vi "FilterSettings.Reset.vi"(8 "error in (no error)":errorcluster, 10 "Default Filter":T1, 11 "FilterDVR.Ref":refnum<data-value>) -> (0 "error out":errorcluster, 3 "Filter":T1)   [LabVIEW 2025, in "bus_monitor_server_do.lvlib"]
uses:
  bus_monitor_server_do.lvlib
  bus_monitor_server/RPC Messages/ni_bus_monitor_api_FilterInfo.ctl
  bus_monitor_server/RPC Messages/ni_bus_monitor_api_DirectionFilter.ctl
  bus_monitor_server/RPC Messages/ni_bus_monitor_api_FrameFilter.ctl
  bus_monitor_server/bus_monitor_server.lvlib
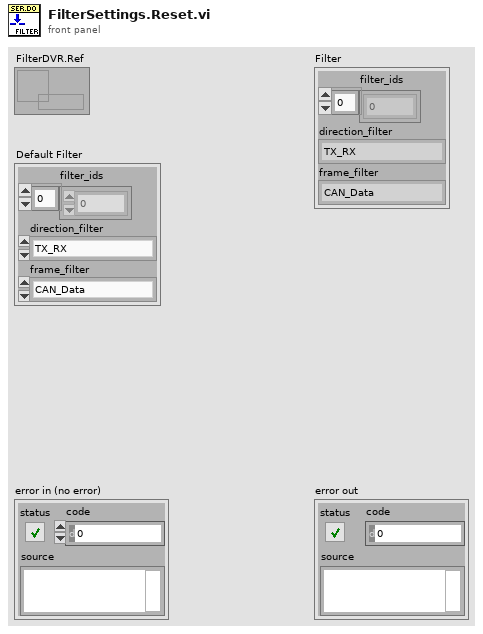
[diagram p1: front panel]
types:
  T1 = typedef "bus_monitor_server.lvlib/ni_bus_monitor_api_FilterInfo.ctl" = cluster{"filter_ids":u32[], "direction_filter":T2, "frame_filter":T3}
  T2 = typedef "bus_monitor_server.lvlib/ni_bus_monitor_api_DirectionFilter.ctl" = enum32{"TX_RX", "RX", "TX"}
  T3 = typedef "bus_monitor_server.lvlib/ni_bus_monitor_api_FrameFilter.ctl" = enum32{"CAN_Data", "CAN_Remote", "CAN_Bus_Error", "CAN_2_Data", "CAN_FD_Data", "CAN_FD_BRS_Data", "J1939_Data", "Delay", "Log_Trigger", "Start_Trigger", "All"}
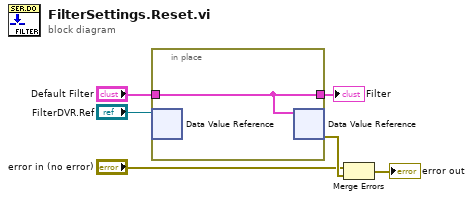
[diagram p0: block diagram]
diagram:
  n1 = in-place {
    in-place-border: "Default Filter" -> [w7]
    in-place-border: [w7] -> w3
    n2 = in-place-dvr #1("FilterDVR.Ref") -> ()  [unwired: 2 out]
    n3 = in-place-dvr #1(w7) -> (w5:errorcluster)  [unwired: 1 out]
  }
  "Filter" <- w3
  n4 = Merge Errors("error in (no error)", w5) -> (→"error out":errorcluster)
